vi "Roller Motor Control.vi"(7 "Action":T1=enum."Off", 8 "Error in":errorcluster, 11 "RelayDevRef":T2={"DevStatus"={"status"=FALSE, "code"=0, "source"=""}, "Relay Channel"=enum."Invalid", "Digital Module"=enum."Digital Module 1", "Relay Direction"=enum."Both directions"}) -> (0 "Error out":errorcluster)   [LabVIEW 2013]
doc: "RollerMotor controls the roller (using a spike relay). It has the following actions:\n-Init: takes a reference to the relay and stores it in a shift register so that it does not have to be passed in again\n-Forward: turns the roller TOWRAD the robot\n-Off: shuts off the roller\n-Reverse: turns the roller AWAY from the robot"
uses:
  <vilib>/Rock Robotics/WPI/Relay/WPI_RelayDevRef.ctl
  <vilib>/Rock Robotics/SystemInterfaces/DIO/FPGA_DIORelayChannel.ctl
  <vilib>/Rock Robotics/SystemInterfaces/Typedef/FPGA_TypedefDigitalModule.ctl
  <vilib>/Rock Robotics/WPI/Relay/WPI_RelayDirection.ctl
  RollerAction.ctl
  <vilib>/Rock Robotics/WPI/Relay/WPI_RelayValue.ctl
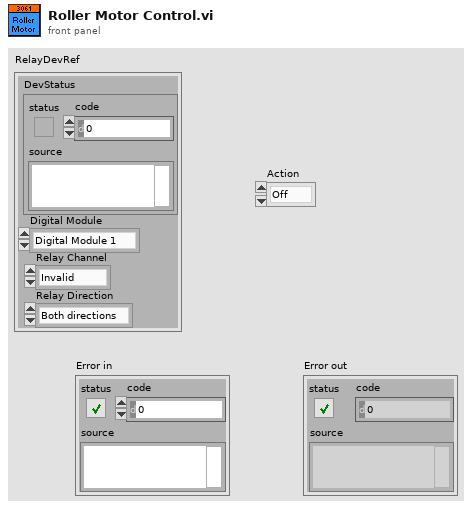
[diagram p1: front panel]
types:
  T1 = typedef "RollerAction.ctl" = enum16{"Init", "Off", "Forward", "Reverse"}
  T2 = typedef "WPI_RelayDevRef.ctl" = cluster{"DevStatus":errorcluster, "Relay Channel":T3, "Digital Module":T4, "Relay Direction":T5}
  T3 = typedef "FPGA_DIORelayChannel.ctl" = enum8{"Relay 1", "Relay 2", "Relay 3", "Relay 4", "Relay 5", "Relay 6", "Relay 7", "Relay 8", "Invalid"}
  T4 = typedef "FPGA_TypedefDigitalModule.ctl" = enum16{"Digital Module 1", "Digital Module 2"}
  T5 = typedef "WPI_RelayDirection.ctl" = enum16{"Both directions", "Forward only", "Reverse only"}
  T6 = typedef "WPI_RelayValue.ctl" = enum16{"Off", "On", "Forward", "Reverse"}
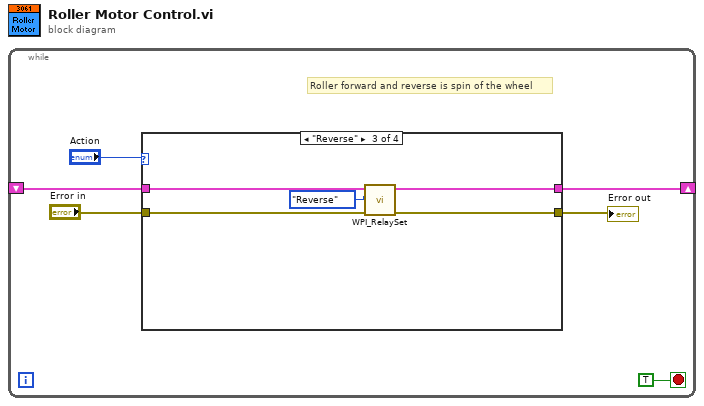
[diagram p0: block diagram]
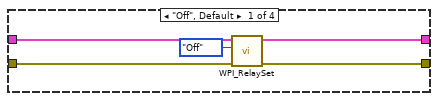
[diagram p2: hidden frame]
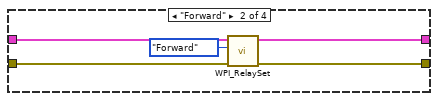
[diagram p3: hidden frame]
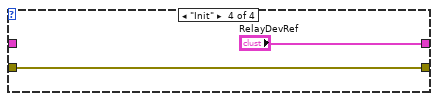
[diagram p4: hidden frame]
diagram:
  n1 = while {
    shift-right: [w4] -> _
    shift-left: _ -> [w3]
    stop <- TRUE stop-if-true
    # "Roller forward and reverse is spin of the wheel"
    n2 = case shown="\"Reverse\"" "Action" {
      tunnel: "Error in" -> [w10 w14 w19 w23]
      tunnel: [w9 w13 w18 w23] -> w1
      tunnel: [w8 w16 w20 "RelayDevRef"] -> w4
      tunnel: w3 -> [w7 w12 w17 _]
      frame "Off", Default {
        n3 = call <vilib>:"WPI_RelaySet.vi"("error in (no error)"=w10, "RelayValue"=WPI_RelayValue."Off", "RelayDevRef"=w7) -> ("error out"=w9:errorcluster, "RelayDevRef"=w8:T2)  [unwired: 7 in]
      }
      frame "Forward" {
        n4 = call <vilib>:"WPI_RelaySet.vi"("error in (no error)"=w14, "RelayValue"=WPI_RelayValue."Forward", "RelayDevRef"=w12) -> ("error out"=w13:errorcluster, "RelayDevRef"=w16:T2)  [unwired: 7 in]
      }
      frame "Reverse" {
        n5 = call <vilib>:"WPI_RelaySet.vi"("error in (no error)"=w19, "RelayValue"=WPI_RelayValue."Reverse", "RelayDevRef"=w17) -> ("error out"=w18:errorcluster, "RelayDevRef"=w20:T2)  [unwired: 7 in]
      }
      frame "Init" {
      }
    }
    "Error out" <- w1
  }
